vi "Monitor.vi"() -> ()   [LabVIEW 2023]
uses:
  instr.lib/Siemens ELAN/Message Header.ctl
  instr.lib/Siemens ELAN/Channel Status.ctl
  instr.lib/Siemens ELAN/Unit Dimensions.ctl
  instr.lib/Siemens ELAN/Measured variables.ctl
  instr.lib/Siemens ELAN/Siemens ELAN.lvlib
panel:
  out "Loop Number":i32
  out "Measured variables":T1[](array[typedef])
  out "Measurements":cluster{"Measured value":dbl, "Dimension":T2}[](array[cluster]) {"Measured value" format="%#_6f"}
  in  "Source Address":u8=208 format="%.0x"
  in  "Target Address":u8=16 format="%.0x"
  in  "New Name":string
  in  "VISA resource name":refnum<visa-resource-name>="ULTRAMAT"
  in  "Set Clock":bool
  in  "VISA Timeout Value":u32=200
  out "Channel Name":string
  in  "Broadcast ON?":bool
  out "Maintenance Requests":T3(array[ring])
  in  "Reset":bool
  in  "Remote ON?":bool
  in  "Maintenance ON?":bool
  out "Faults/Errors":T4(array[ring])
  out "time stamp":timestamp format="%<%Y-%m-%dT%H:%M:%S>T"
  out "Channel":T5
  out "Channel Type":T6(ring)
  out "x-y":u32
  in  "milliseconds to wait":u32
  in  "stop":bool
  out "Success":bool
  out "Message Header":T7 {"Source Address" format="%.0x"; "Target Address" format="%.0x"}
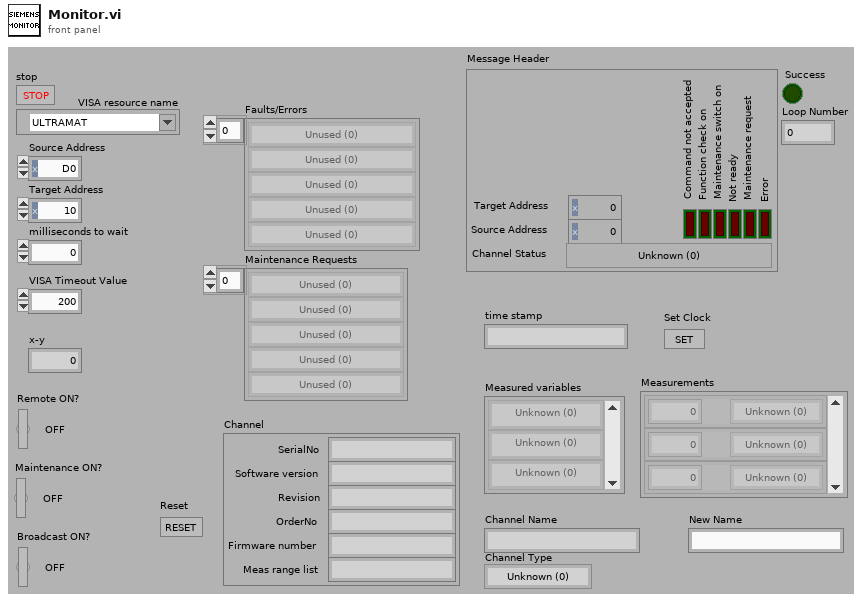
[diagram p1: front panel]
types:
  T1 = typedef "Siemens ELAN.lvlib/Measured variables.ctl" = enum8{"Unknown (0)", "No component", "CO", "CO2", "CH4", "C6H14", "SO2", "NO", "NO2", "CHClF2 (R22)", "C3H8", "C4H10", "O2", "C5H12", "HC", "Pressure", "pH", "Temperature", "C2H4", "C2H2", "C3H6", "C4H6", "C4H8", "C2H6", "NH3", "N2O", "C6H6", "SF6", "CH3OH", "C2H5OH", "CH2Cl2", "C2H4Cl2", "CH3Cl", "C2H4O", "H2O (vapor)", "G/l", "Unknown (36)", "Unknown (37)", "Unknown (38)", "Unknown (39)", "Unknown (40)", "Unknown (41)", "Unknown (42)", "Unknown (43)", "Unknown (44)", "Unknown (45)", "Unknown (46)", "Unknown (47)", "Unknown (48)", "Unknown (49)", "Unknown (50)", "Unknown (51)", "Unknown (52)", "Unknown (53)", "Unknown (54)", "Unknown (55)", "Unknown (56)", "Unknown (57)", "Unknown (58)", "Unknown (59)", "Unknown (60)", "Unknown (61)", "Unknown (62)", "Unknown (63)", "Unknown (64)", "Unknown (65)", "Unknown (66)", "Unknown (67)", "Unknown (68)", "Unknown (69)", "Unknown (70)", "Unknown (71)", "Unknown (72)", "Unknown (73)", "Unknown (74)", "Unknown (75)", "Unknown (76)", "Unknown (77)", "Unknown (78)", "Unknown (79)", "Unknown (80)", "Unknown (81)", "Unknown (82)", "Unknown (83)", "Unknown (84)", "Unknown (85)", "Unknown (86)", "Unknown (87)", "Unknown (88)", "Unknown (89)", "Unknown (90)", "Unknown (91)", "Unknown (92)", "Unknown (93)", "Unknown (94)", "Unknown (95)", "Unknown ((96)", "Unknown (97)", "Unknown (98)", "Unknown (99)", "Ambient Pressure", "Unknown (>100)"}
  T2 = typedef "Siemens ELAN.lvlib/Unit Dimensions.ctl" = enum8{"Unknown (0)", "Pure number", "ppm", "ppb", "vpm", "vpm C1", "vpm C3", "vpm C6", "mg C/m^3", "mg/m^3", "%", "% v/v", "% of range", "% saturation", "%/°C", "%/K", "% w/w", "mV/pH", "mV/mbar", "nA/mbar", "S/m", "S/cm", "mS/m", "mS/cm", "uS/m", "uS/cm", "s", "min", "hr", "pA", "mA", "uV", "mV", "V", "mbar", "hPa", "ml/min", "kohm", "MOhm", "S", "°C", "Hz", "pH", "ug/l", "mg/l", "l/min", "uA", "mg/dm^3", "kPa", "kohm*cm", "MOhm*cm", "°", "Unknown (>51)"}
  T3 = enum8{"Unused (0)", "Cal Tolerance Violated", "Signal Too High With Zero Adj", "Signal Too Low With Span", "Set Clock", "Microflow Sensor Drift", "Display Temperature", "Analyzer Temperature", "Measuring Head Temperature", "External Request"}[]
  T4 = enum8{"Unused (0)", "Param Memory", "Chopper/Magnetic Field", "Microflow Sensor", "External Fault", "AnalyzerTemperature", "Field Device Heater", "Measuring Head Temperature", "Pressure Sensor", "Signal Too Large", "Unused (S10)", "Reference Gas Supply", "Main Power", "Unused (S13)", "Measured Value > Full Scale", "Calibration Aborted", "Low Sample Flow "}[]
  T5 = cluster{"SerialNo":string, "Software version":string, "Revision":string, "OrderNo":string, "Firmware number":string, "Meas range list":string}
  T6 = enum8{"Unknown (0)", "ULTRAMAT 6", "OXYMAT 6", "FIDAMAT 6", "ULTRAMAT 23", "SIPAN 34", "Unknown (6)", "CALOMAT 6", "Unknown (>7)"}
  T7 = typedef "Siemens ELAN.lvlib/Message Header.ctl" = cluster{"Target Address":u8, "Source Address":u8, "Error":bool, "Maintenance request":bool, "Not ready":bool, "Maintenance switch on":bool, "Function check on":bool, "Command not accepted":bool, "Channel Status":T8}
  T8 = typedef "Siemens ELAN.lvlib/Channel Status.ctl" = enum8{"Unknown (0)", "Warm-up", "Pause", "Standby", "Measure", "Zero calibration", "Adjust component slope", "Unknown (7)", "Adjust curve dip", "Adjust linearization sensitivity", "Adjust temperature compensation", "Adjust pressure compensation", "Adjust linearization zero", "Adjust flow sensor", "Autocal", "Adjust phase", "Zero calibration of O2 sensor", "Synchronous zero calibration", "Purging for synchronous zero calibration", "Adjust analog output", "Adjust analog input", "Cleaning", "Unknown (>21)"}
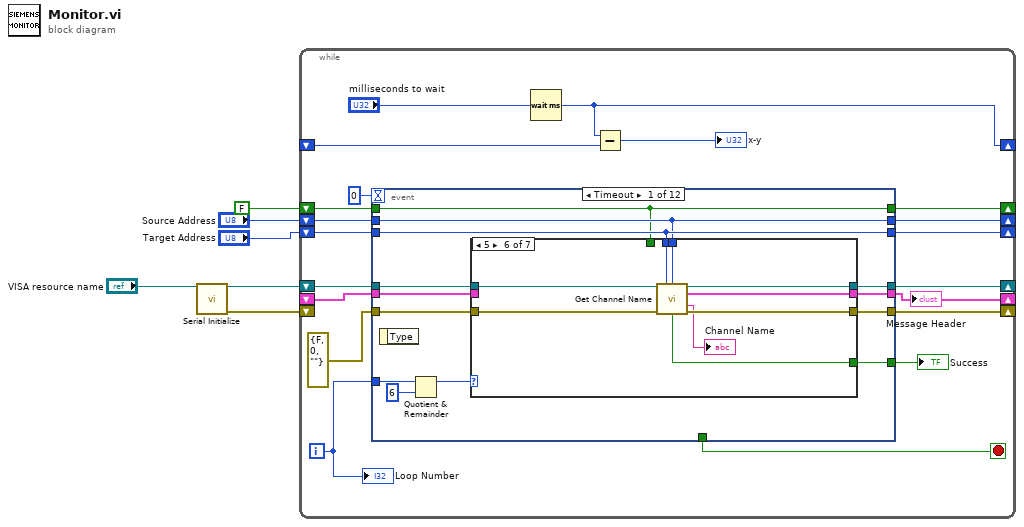
[diagram p0: block diagram]
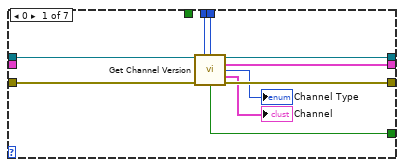
[diagram p2: hidden frame]
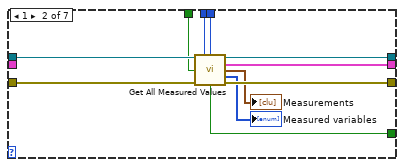
[diagram p3: hidden frame]
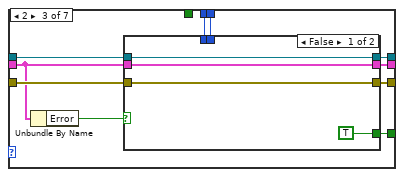
[diagram p4: hidden frame]
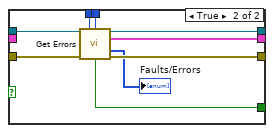
[diagram p5: hidden frame]
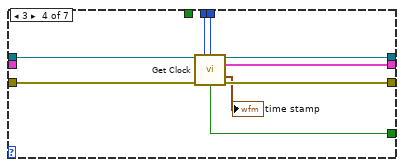
[diagram p6: hidden frame]
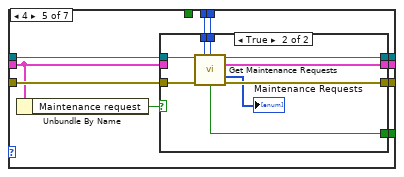
[diagram p7: hidden frame]
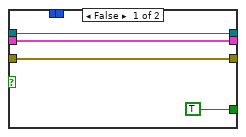
[diagram p8: hidden frame]
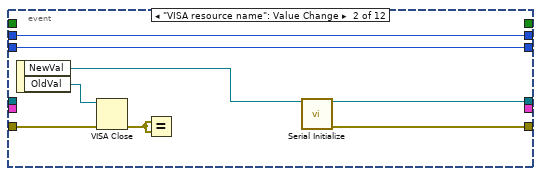
[diagram p10: hidden frame]
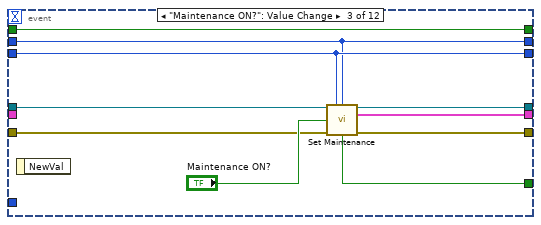
[diagram p11: hidden frame]
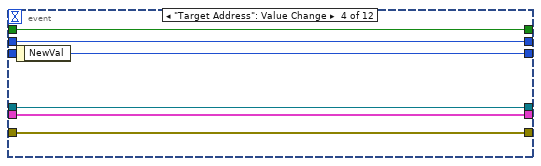
[diagram p12: hidden frame]
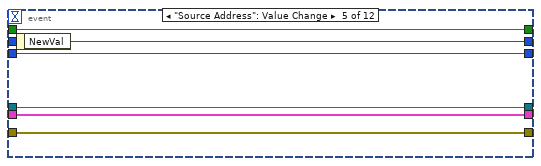
[diagram p13: hidden frame]
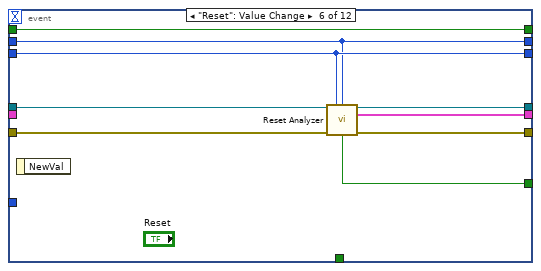
[diagram p14: hidden frame]
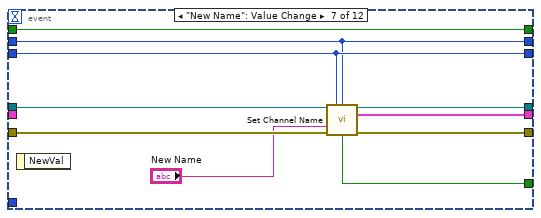
[diagram p15: hidden frame]
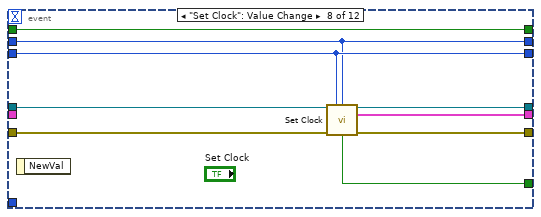
[diagram p16: hidden frame]
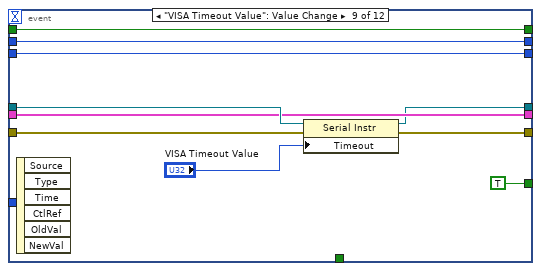
[diagram p17: hidden frame]
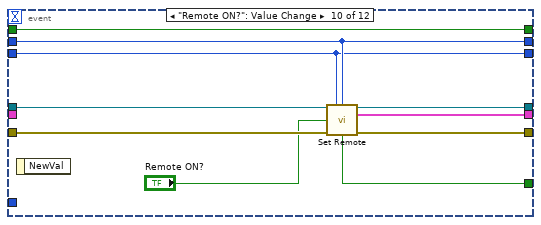
[diagram p18: hidden frame]
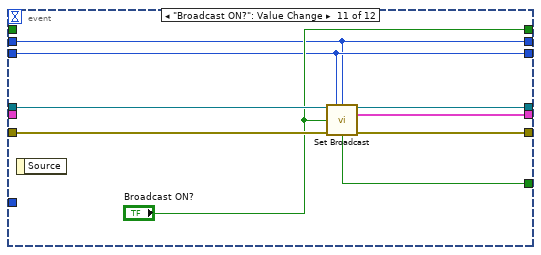
[diagram p19: hidden frame]
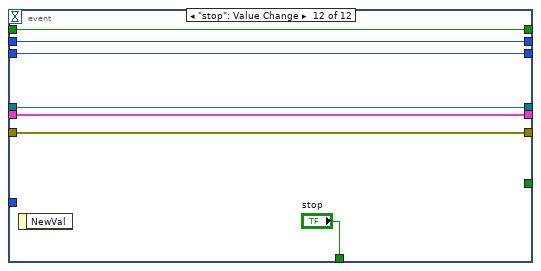
[diagram p20: hidden frame]
diagram:
  n1 = call "Serial Initialize.vi"("VISA Session In"="VISA resource name") -> ("VISA Session Out"=w2:refnum<visa-resource-name>, "error out"=w1:errorcluster)  [unwired: 13 in]
  n2 = while {
    shift-right: [w20] -> _
    shift-left: w2 -> [w22]
    shift-right: [w21] -> _
    shift-left: w1 -> [_]
    shift-right: [w26] -> _
    shift-left: _ -> [w25]
    shift-right: [w16] -> _
    shift-left: _ -> [w15]
    shift-right: [w13] -> _
    shift-left: FALSE -> [w14]
    shift-right: [w10] -> _
    shift-left: "Source Address" -> [w12]
    shift-right: [w9] -> _
    shift-left: "Target Address" -> [w11]
    i -> [w7]
    stop <- w8 stop-if-true
    n3 = event shown="[0] Timeout" {
      selector: _ -> [_ _ _ _ _ _ _ _ _ _ _ _]
      dyn-events: _ -> [_ _ _ _ _ _ _ _ _ _ _ _]
      timeout: 0 -> [_ _ _ _ _ _ _ _ _ _ _ _]
      tunnel: w22 -> [w36 _ w144 w150 w156 w166 w176 w185 w194 w205 w214 w220]
      tunnel: errorcluster {"status"=FALSE, "code"=0, "source"=""} ("error out") -> [w34 w128 w143 w149 w155 w165 w175 w184 w191 w204 w213 w219]
      tunnel: [w33 w132 w141 w149 w155 w162 w172 w181 w189 w201 w211 w219] -> w21
      tunnel: [w35 w133 w142 w150 w156 w164 w174 w183 w190 w203 w212 w220] -> w20
      tunnel: [_ _ _ _ _ _ _ _ _ _ _ "stop"] -> w8
      tunnel: w7 -> [w39 _ _ _ _ _ _ _ _ _ _ _]
      tunnel: [w32 _ w140 w148 w154 w163 w173 w182 w193 w202 w210 w218] -> w16
      tunnel: [w31 _ w139 _ _ w161 w171 w180 TRUE ("Success") w200 w209 _] -> w18
      tunnel: w15 -> [w30 _ _ w148 w154 _ _ _ w193 _ _ w218]
      tunnel: [w27 _ w138 w151 w157 w160 w170 w179 w195 w198 "Broadcast ON?" w217] -> w13
      tunnel: w14 -> [w27 _ w138 w151 w157 w160 w170 w179 w195 w198 _ w217]
      tunnel: w12 -> [w28 w135 w136 w147 _ w158 w167 w177 w186 w197 w206 w215]
      tunnel: w11 -> [w29 w134 w137 _ w152 w159 w168 w178 w187 w196 w207 w216]
      tunnel: [w28 w135 w136 w147 w153 w158 w167 w177 w186 w197 w206 w215] -> w10
      tunnel: [w29 w134 w137 w146 w152 w159 w168 w178 w187 w196 w207 w216] -> w9
      event Timeout {
        n4 = event-data() -> ()  [unwired: 1 in, 1 out]
        n5 = Quotient & Remainder(x=w39, y=6) -> (x-y*floor(x/y)=w37:i32)  [unwired: 1 out]
        n6 = case shown="5" w37 {
          tunnel: w36 -> [w47 w60 w68 w92 w102 w124 w127]
          tunnel: [w46 w59 w67 w89 w100 w122 w127] -> w35
          tunnel: w34 -> [w45 w58 w70 w91 w101 w123 w126]
          tunnel: [w49 w57 w69 w90 w98 w120 w126] -> w33
          tunnel: [w44 w56 w66 w87 w99 w121 w125] -> w32
          tunnel: [w43 w55 w65 w86 w97 w119 _] -> w31
          tunnel: w30 -> [_ _ w63 _ w95 _ w125]
          tunnel: w29 -> [w41 w54 w62 w85 w94 w117 _]
          tunnel: w28 -> [w40 w53 w61 w84 w93 w116 _]
          tunnel: w27 -> [_ w50 _ _ _ _ _]
          frame 0 {
            n7 = call "Get Channel Version.vi"("VISA Session In"=w47, "Target Address"=w41, "Source Address"=w40, "error in (no error)"=w45) -> ("VISA Session Out"=w46:refnum<visa-resource-name>, "Message Header"=w44:T7, "Channel Type"=→"Channel Type":T6, "Channel"=→"Channel":T5, "Success"=w43:bool, "error out"=w49:errorcluster)  [unwired: 6 in]
          }
          frame 1 {
            n8 = call "Get All Measured Values.vi"("VISA Session In"=w60, "Target Address"=w54, "Source Address"=w53, "Use Broadcast?(F)"=w50, "error in (no error)"=w58) -> ("VISA Session Out"=w59:refnum<visa-resource-name>, "Message Header"=w56:T7, "Measurements"=→"Measurements":cluster{"Measured value":dbl, "Dimension":T2}[], "Measured variables"=→"Measured variables":T1[], "Success"=w55:bool, "error out"=w57:errorcluster)  [unwired: 5 in]
          }
          frame 2 {
            n9 = Unbundle By Name(w63) -> ("Error"=w64:bool)
            n10 = case shown="False" w64 {
              tunnel: w70 -> [w74 w83]
              tunnel: [w74 w82] -> w69
              tunnel: w68 -> [w72 w81]
              tunnel: [w72 w80] -> w67
              tunnel: [w73 w79] -> w66
              tunnel: [TRUE ("Success") w77] -> w65
              tunnel: w63 -> [w73 _]
              tunnel: w62 -> [_ w76]
              tunnel: w61 -> [_ w75]
              frame False {
              }
              frame True {
                n11 = call "Get Errors.vi"("VISA Session In"=w81, "Target Address"=w76, "Source Address"=w75, "error in (no error)"=w83) -> ("VISA Session Out"=w80:refnum<visa-resource-name>, "Message Header"=w79:T7, "Faults/Errors"=→"Faults/Errors":T4, "Success"=w77:bool, "error out"=w82:errorcluster)  [unwired: 7 in]
              }
            }
          }
          frame 3 {
            n12 = call "Get Clock.vi"("VISA Session In"=w92, "Target Address"=w85, "Source Address"=w84, "error in (no error)"=w91) -> ("VISA Session Out"=w89:refnum<visa-resource-name>, "Message Header"=w87:T7, "time stamp"=→"time stamp":timestamp, "Success"=w86:bool, "error out"=w90:errorcluster)  [unwired: 7 in]
          }
          frame 4 {
            n13 = Unbundle By Name(w95) -> ("Maintenance request"=w96:bool)
            n14 = case shown="True" w96 {
              tunnel: w102 -> [w105 w115]
              tunnel: w101 -> [w106 w114]
              tunnel: [w105 w113] -> w100
              tunnel: [w104 w112] -> w99
              tunnel: [w106 w111] -> w98
              tunnel: [TRUE ("Success") w110] -> w97
              tunnel: w95 -> [w104 _]
              tunnel: w94 -> [_ w108]
              tunnel: w93 -> [_ w107]
              frame False {
              }
              frame True {
                n15 = call "Get Maintenance Requests.vi"("VISA Session In"=w115, "Target Address"=w108, "Source Address"=w107, "error in (no error)"=w114) -> ("VISA Session Out"=w113:refnum<visa-resource-name>, "Message Header"=w112:T7, "Maintenance Requests"=→"Maintenance Requests":T3, "Success"=w110:bool, "error out"=w111:errorcluster)  [unwired: 7 in]
              }
            }
          }
          frame 5 {
            n16 = call "Get Channel Name.vi"("VISA Session In"=w124, "Target Address"=w117, "Source Address"=w116, "error in (no error)"=w123) -> ("VISA Session Out"=w122:refnum<visa-resource-name>, "Message Header"=w121:T7, "Channel Name"=→"Channel Name":string, "Success"=w119:bool, "error out"=w120:errorcluster)  [unwired: 7 in]
          }
          frame Default {
          }
        }
      }
      event "VISA resource name": Value Change {
        n17 = event-data() -> ("NewVal"=w131:refnum<visa-resource-name>, "OldVal"=w130:refnum<visa-resource-name>)  [unwired: 1 in]
        n18 = VISA Close(VISA resource name=w130, error in (no error)=w128) -> (error out=w129:errorcluster)
        n19 = Equal?(x=w129, y=w129) -> ()  [unwired: 1 out]
        n20 = call "Serial Initialize.vi"("VISA Session In"=w131) -> ("VISA Session Out"=w133:refnum<visa-resource-name>, "error out"=w132:errorcluster)  [unwired: 13 in]
      }
      event "Maintenance ON?": Value Change {
        n21 = event-data() -> ()  [unwired: 1 in, 1 out]
        n22 = call "Set Maintenance.vi"("VISA Session In"=w144, "Target Address"=w137, "Source Address"=w136, "Maintenance ON?"="Maintenance ON?", "error in (no error)"=w143) -> ("VISA Session Out"=w142:refnum<visa-resource-name>, "Message Header"=w140:T7, "Success"=w139:bool, "error out"=w141:errorcluster)  [unwired: 7 in]
      }
      event "Target Address": Value Change {
        n23 = event-data() -> ("NewVal"=w146:u8)  [unwired: 1 in]
      }
      event "Source Address": Value Change {
        n24 = event-data() -> ("NewVal"=w153:u8)  [unwired: 1 in]
      }
      event "Reset": Value Change {
        n25 = event-data() -> ()  [unwired: 1 in, 1 out]
        n26 = call "Reset Analyzer.vi"("VISA Session In"=w166, "Target Address"=w159, "Source Address"=w158, "error in (no error)"=w165) -> ("VISA Session Out"=w164:refnum<visa-resource-name>, "Message Header"=w163:T7, "Success"=w161:bool, "error out"=w162:errorcluster)  [unwired: 8 in]
      }
      event "New Name": Value Change {
        n27 = event-data() -> ()  [unwired: 1 in, 1 out]
        n28 = call "Set Channel Name.vi"("VISA Session In"=w176, "Target Address"=w168, "Source Address"=w167, "Channel Name"="New Name", "error in (no error)"=w175) -> ("VISA Session Out"=w174:refnum<visa-resource-name>, "Message Header"=w173:T7, "Success"=w171:bool, "error out"=w172:errorcluster)  [unwired: 7 in]
      }
      event "Set Clock": Value Change {
        n29 = event-data() -> ()  [unwired: 1 in, 1 out]
        n30 = call "Set Clock.vi"("VISA Session In"=w185, "Target Address"=w178, "Source Address"=w177, "error in (no error)"=w184) -> ("VISA Session Out"=w183:refnum<visa-resource-name>, "Message Header"=w182:T7, "Success"=w180:bool, "error out"=w181:errorcluster)  [unwired: 8 in]
      }
      event "VISA Timeout Value": Value Change {
        n31 = event-data() -> ()  [unwired: 1 in, 6 out]
        n32 = property class="Serial Instr"(reference=w194, error in=w191, "Timeout"="VISA Timeout Value") -> (reference out=w190:refnum<visa-resource-name>, error out=w189:errorcluster)
      }
      event "Remote ON?": Value Change {
        n33 = event-data() -> ()  [unwired: 1 in, 1 out]
        n34 = call "Set Remote.vi"("VISA Session In"=w205, "Target Address"=w196, "Source Address"=w197, "Remote ON?"="Remote ON?", "error in (no error)"=w204) -> ("VISA Session Out"=w203:refnum<visa-resource-name>, "Message Header"=w202:T7, "Success"=w200:bool, "error out"=w201:errorcluster)  [unwired: 7 in]
      }
      event "Broadcast ON?": Value Change {
        n35 = event-data() -> ()  [unwired: 1 in, 1 out]
        n36 = call "Set Broadcast.vi"("VISA Session In"=w214, "Target Address"=w207, "Source Address"=w206, "Broadcast ON?"="Broadcast ON?", "error in (no error)"=w213) -> ("VISA Session Out"=w212:refnum<visa-resource-name>, "Message Header"=w210:T7, "Success"=w209:bool, "error out"=w211:errorcluster)  [unwired: 7 in]
      }
      event "stop": Value Change {
        n37 = event-data() -> ()  [unwired: 1 in, 1 out]
      }
    }
    "Message Header" <- w16
    "Success" <- w18
    n38 = Wait (ms)(milliseconds to wait="milliseconds to wait") -> (millisecond timer value=w26:u32)
    n39 = Subtract(x=w26, y=w25) -> (x-y=→"x-y":u32)
    "Loop Number" <- w7
  }
